vi "test Get-Set-Get Default Word Value.vi"(8 "error in":errorcluster, 11 "TestCase in":refnum<class "Scripting.lvclass">) -> (0 "error out":errorcluster, 3 "TestCase out":refnum<class "Scripting.lvclass">)   [LabVIEW 2020, in "Scripting.lvclass"]
uses:
  Scripting.lvclass
  Shared/VS Channels Definition for Label.ctl
  Shared/VS Channel Definition for Parameter.ctl
  Shared/Parameter Definition.ctl
  <vilib>/NI/NI VeriStand Encoding and Decoding/Encoding.ctl
  Shared/Transfer Type.ctl
  Shared/Direction.ctl
  Scripting.lvclass/Scripting.ctl
  <vilib>/addons/_JKI Toolkits/VI Tester/TestCase.llb/TestCase.lvclass
  Scripting/AIM/AIM ARINC 429 Scripting.lvlib
  Scripting/ARINC 429/ARINC 429 Scripting.lvlib
  <vilib>/NI/NI VeriStand Encoding and Decoding/Encoding and Decoding.lvlib
  C:/Program Files (x86)/National Instruments/LabVIEW 2020/vi.lib/addons/_JKI Toolkits/VI Tester/TestCase.llb/TestCase.lvclass
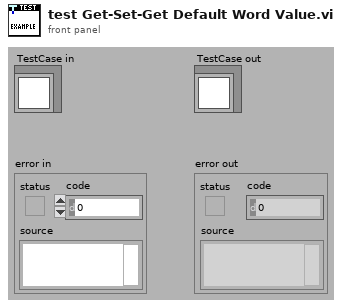
[diagram p1: front panel]
types:
  T1 = typedef "Direction.ctl" = enum16{"Rx", "Tx"}
  T2 = typedef "VS Channels Definition for Label.ctl" = cluster{"label (Dec)":u32, "parameters":T3[], "SDI value":u8, "SDI enabled":bool, "transfer type":T6, "create timestamp":bool}
  T3 = typedef "VS Channel Definition for Parameter.ctl" = cluster{"name":string, "default value":dbl, "unit":string, "Parameter":T4}
  T4 = typedef "Parameter Definition.ctl" = cluster{"start index":i32, "size":i32, "encoding":T5, "signed":bool, "scale multiplier":dbl, "scale offset":dbl}
  T5 = typedef "Encoding and Decoding.lvlib/Encoding.ctl" = enum16{"BNR", "BCD", "Discrete"}
  T6 = typedef "Transfer Type.ctl" = enum16{"Scheduled", "Acyclic", "Block", "Strobe"}
  T7 = typedef "Custom Device API.lvlib/Custom Device Item Ref.ctl" = u64
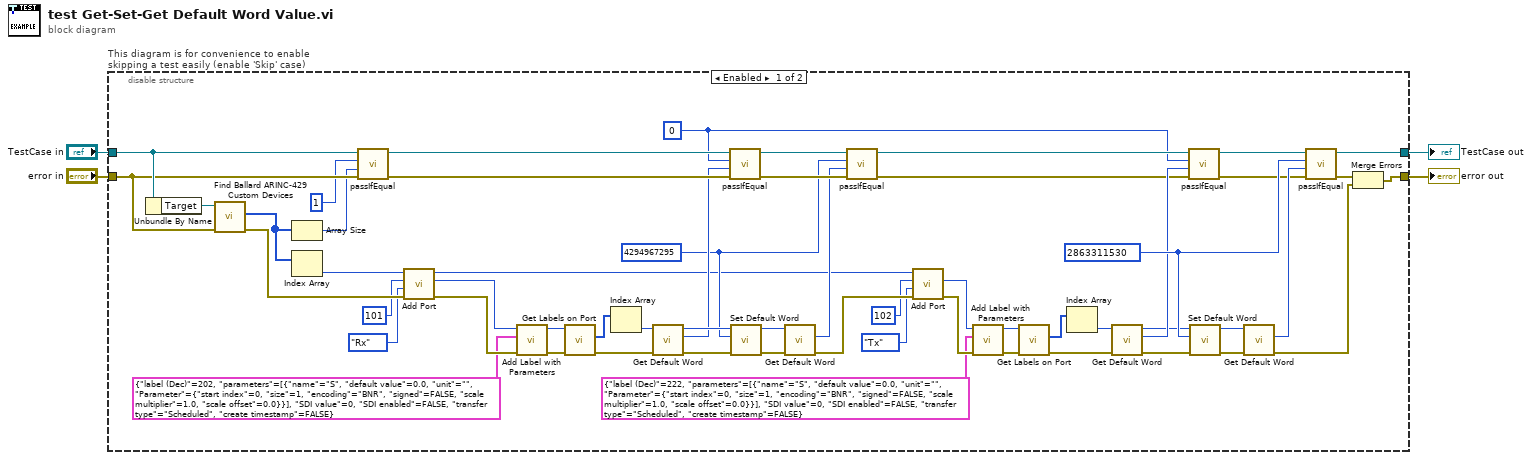
[diagram p0: block diagram]
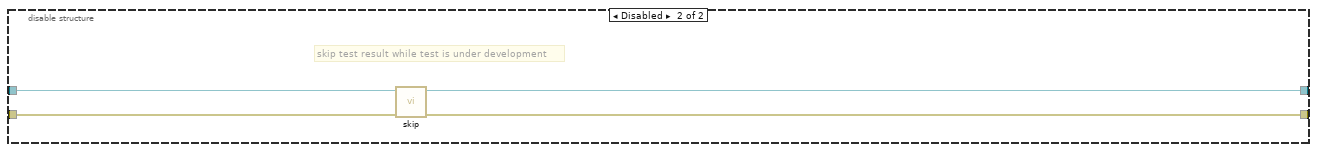
[diagram p2: hidden frame]
diagram:
  n1 = disable-structure "This diagram is for convenience to enable skipping a test easily (enable 'Skip' case)" shown="Enabled" {
    disable-tunnel: "TestCase in" -> [w60 w65]
    disable-tunnel: [w25 w63] -> w1
    disable-tunnel: [w56 w64] -> w3
    disable-tunnel: "error in" -> [w59 w62]
    frame Enabled {
      w39 = u32 2863311530 ("default word")
      w42 = u32 4294967295 ("default word")
      w24 = u32 0 ("default word")
      n2 = Unbundle By Name(w60) -> ("Target"=w61:refnum<k24>)
      n3 = call "Find Ballard ARINC-429 Custom Devices.vi"("error in"=w59, "target in"=w61) -> ("error out"=w21:errorcluster, "AIM ARINC 429 custom devices"=w23:u64[])  [unwired: 7 in, 1 out]
      n4 = Array Size(array=w23) -> (size(s)=w57:i32)
      n5 = Index Array(array=w23) -> (element=w22:u64)  [unwired: 1 in]
      n6 = call-dynamic "passIfEqual.vi"("error in (no error)"=w59, "y"=w57, "x"=1 ("size(s)"), "TestCase in"=w60) -> ("error out"=w46:errorcluster, "TestCase out"=w47:refnum<class "Scripting.lvclass">)  [unwired: 6 in]
      n7 = call "Add Port.vi"("error in"=w21, "direction"=Direction."Rx", "port number"=u16 101, "AIM ARINC 429 custom device in"=w22) -> ("error out"=w15:errorcluster, "port"=w16:T7, "AIM ARINC 429 custom device out"=w19:T7)  [unwired: 5 in]
      n8 = call "Add Label with Parameters.vi"("error in"=w15, "label"=T2 {"label (Dec)"=202, "parameters"=[{"name"="S", "default value"=0.0, "unit"="", "Parameter"={"start index"=0, "size"=1, "encoding"=enum."BNR", "signed"=FALSE, "scale multiplier"=1.0, "scale offset"=0.0}}], "SDI value"=0, "SDI enabled"=FALSE, "transfer type"=enum."Scheduled", "create timestamp"=FALSE}, "port ref"=w16) -> ("error out"=w13:errorcluster, "port ref out"=w12:T7)  [unwired: 7 in]
      n9 = call "Get Labels on Port.vi"("error in"=w13, "port in"=w12) -> ("error out"=w53:errorcluster, "labels"=w54:T7[])  [unwired: 6 in, 2 out]
      n10 = Index Array(array=w54) -> (element=w52:T7)  [unwired: 1 in]
      n11 = call "Get Default Word.vi"("error in"=w53, "Item Ref in"=w52) -> ("error out"=w51:errorcluster, "default word"=w45:u32, "Item Ref out"=w50:T7)  [unwired: 7 in]
      n12 = call-dynamic "passIfEqual.vi"("error in (no error)"=w46, "y"=w45, "x"=w24, "TestCase in"=w47) -> ("error out"=w43:errorcluster, "TestCase out"=w44:refnum<class "Scripting.lvclass">)  [unwired: 6 in]
      n13 = call "Set Default Word.vi"("error in"=w51, "default word"=w42, "label ref in"=w50) -> ("error out"=w49:errorcluster, "label ref out"=w48:T7)  [unwired: 7 in]
      n14 = call "Get Default Word.vi"("error in"=w49, "Item Ref in"=w48) -> ("error out"=w18:errorcluster, "default word"=w41:u32)  [unwired: 7 in, 1 out]
      n15 = call-dynamic "passIfEqual.vi"("error in (no error)"=w43, "y"=w41, "x"=w42, "TestCase in"=w44) -> ("error out"=w32:errorcluster, "TestCase out"=w28:refnum<class "Scripting.lvclass">)  [unwired: 6 in]
      n16 = call "Add Port.vi"("error in"=w18, "direction"=Direction."Tx", "port number"=u16 102, "AIM ARINC 429 custom device in"=w19) -> ("error out"=w10:errorcluster, "port"=w11:T7)  [unwired: 5 in, 1 out]
      n17 = call "Add Label with Parameters.vi"("error in"=w10, "label"=T2 {"label (Dec)"=222, "parameters"=[{"name"="S", "default value"=0.0, "unit"="", "Parameter"={"start index"=0, "size"=1, "encoding"=enum."BNR", "signed"=FALSE, "scale multiplier"=1.0, "scale offset"=0.0}}], "SDI value"=0, "SDI enabled"=FALSE, "transfer type"=enum."Scheduled", "create timestamp"=FALSE}, "port ref"=w11) -> ("error out"=w8:errorcluster, "port ref out"=w9:T7)  [unwired: 7 in]
      n18 = call "Get Labels on Port.vi"("error in"=w8, "port in"=w9) -> ("error out"=w31:errorcluster, "labels"=w55:T7[])  [unwired: 6 in, 2 out]
      n19 = Index Array(array=w55) -> (element=w30:T7)  [unwired: 1 in]
      n20 = call "Get Default Word.vi"("error in"=w31, "Item Ref in"=w30) -> ("error out"=w33:errorcluster, "default word"=w37:u32, "Item Ref out"=w34:T7)  [unwired: 7 in]
      n21 = call-dynamic "passIfEqual.vi"("error in (no error)"=w32, "y"=w37, "x"=w24, "TestCase in"=w28) -> ("error out"=w38:errorcluster, "TestCase out"=w27:refnum<class "Scripting.lvclass">)  [unwired: 6 in]
      n22 = call "Set Default Word.vi"("error in"=w33, "default word"=w39, "label ref in"=w34) -> ("error out"=w35:errorcluster, "label ref out"=w36:T7)  [unwired: 7 in]
      n23 = call "Get Default Word.vi"("error in"=w35, "Item Ref in"=w36) -> ("error out"=w29:errorcluster, "default word"=w40:u32)  [unwired: 7 in, 1 out]
      n24 = call-dynamic "passIfEqual.vi"("error in (no error)"=w38, "y"=w40, "x"=w39, "TestCase in"=w27) -> ("error out"=w26:errorcluster, "TestCase out"=w25:refnum<class "Scripting.lvclass">)  [unwired: 6 in]
      n25 = Merge Errors(w26, w29) -> (w56:errorcluster)
    }
    frame Disabled {
      # "skip test result while test is under development"
      n26 = call <vilib>:"skip.vi"("error in (no error)"=w62, "TestCase in"=w65) -> ("error out"=w64:errorcluster, "TestCase out"=w63:refnum<class "Scripting.lvclass">)  [unwired: 8 in]
    }
  }
  "error out" <- w3
  "TestCase out" <- w1
